vi "Global Variables.vi"() -> ()   [LabVIEW 2015]
uses:
  Arm Mode TypeDef.ctl
  Arm Notifier TypeDef.ctl
  Operator-Interface-Control-Board.git/trunk/LabVIEW/Analog_Input_TypeDef.ctl
  Operator-Interface-Control-Board.git/trunk/LabVIEW/Switch_Input_TypeDef.ctl
  Arm Mode LEDs.ctl
  IMU AHRS TypeDef.ctl
  Autonomous Mode.ctl
panel:
  in  "Arm Manual Angle":dbl
  in  "Autonomous Mode":T1
  out "Distance (cm)":dbl
  out "Arm Angle":dbl
  in  "Reset IMU":bool
  out "IMU Calibrated":bool
  in  "IMU AHRS":T2
  in  "Arm Mode LEDs":T3
  out "Air Pressure":dbl
  in  "Fire Ready":bool
  in  "Switch Inputs":T4
  out "Analog Inputs":T5
  in  "Arm Control":T6={"Arm Mode"=enum."Manual", "Manual Arm Angle"=0.0}
  in  "Current Arm Mode":T7=enum."Manual"
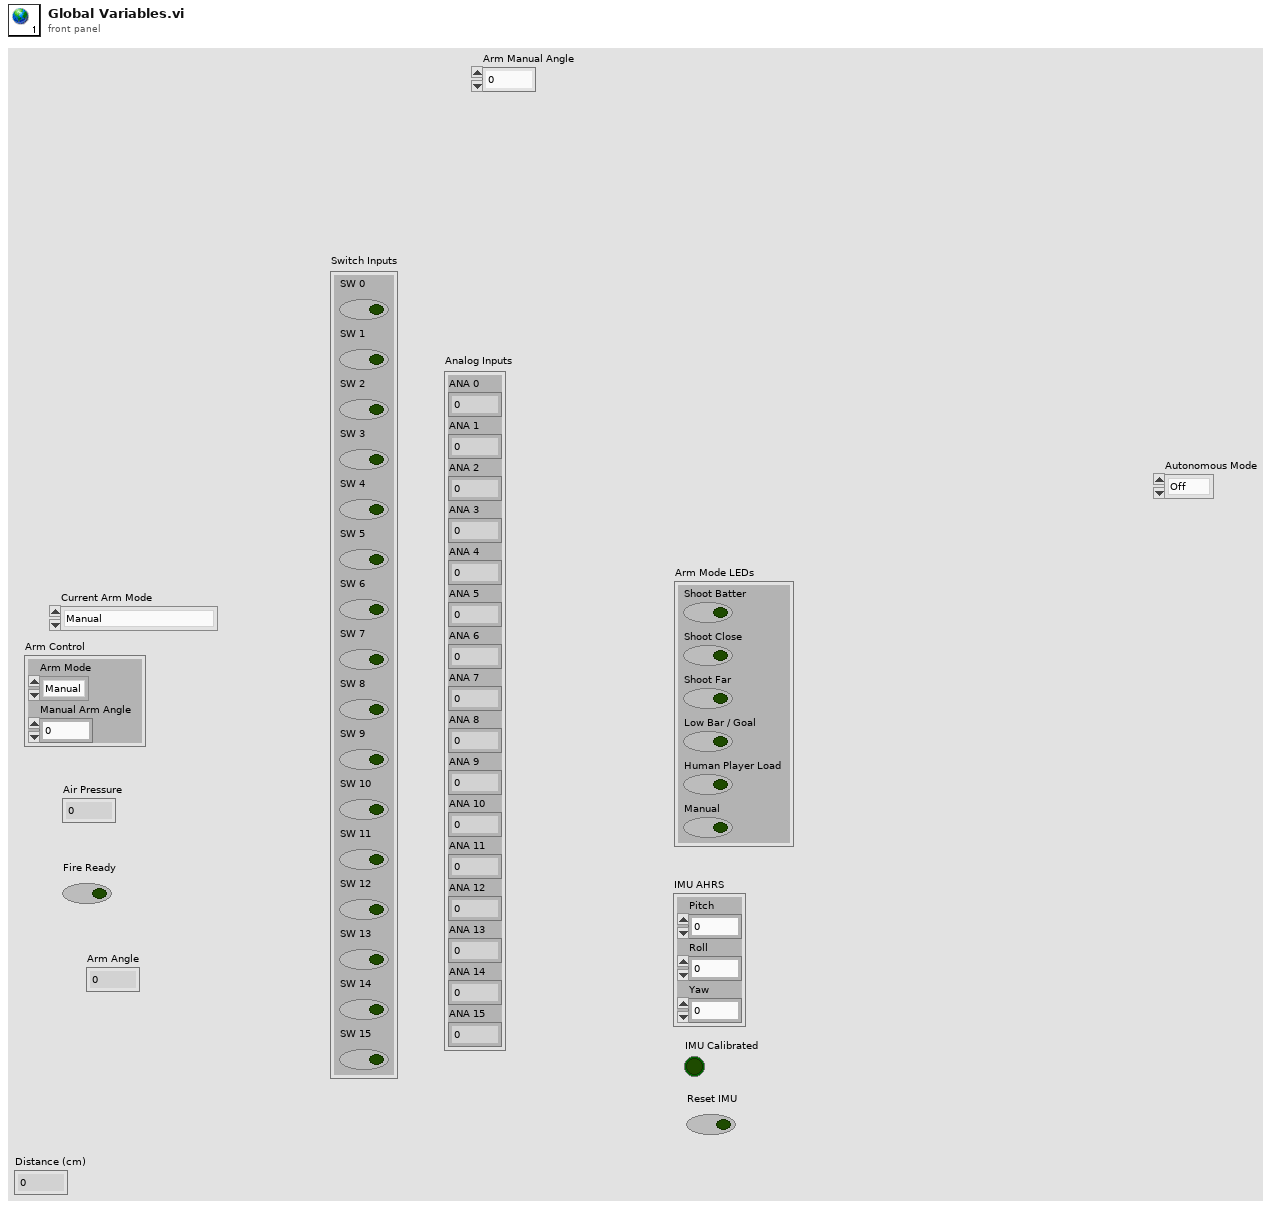
[diagram p1: front panel]
types:
  T1 = typedef "Autonomous Mode.ctl" = enum16{"Off", "Cross Defense", "Shoot A/B", "Shoot C/D", "Shoot E"}
  T2 = typedef "IMU AHRS TypeDef.ctl" = cluster{"Pitch":dbl, "Roll":dbl, "Yaw":dbl}
  T3 = typedef "Arm Mode LEDs.ctl" = cluster{"Shoot Batter":bool, "Shoot Close":bool, "Shoot Far":bool, "Low Bar / Goal":bool, "Human Player Load":bool, "Manual":bool}
  T4 = typedef "Switch_Input_TypeDef.ctl" = cluster{"SW 0":bool, "SW 1":bool, "SW 2":bool, "SW 3":bool, "SW 4":bool, "SW 5":bool, "SW 6":bool, "SW 7":bool, "SW 8":bool, "SW 9":bool, "SW 10":bool, "SW 11":bool, "SW 12":bool, "SW 13":bool, "SW 14":bool, "SW 15":bool}
  T5 = typedef "Analog_Input_TypeDef.ctl" = cluster{"ANA 0":u8, "ANA 1":u8, "ANA 2":u8, "ANA 3":u8, "ANA 4":u8, "ANA 5":u8, "ANA 6":u8, "ANA 7":u8, "ANA 8":u8, "ANA 9":u8, "ANA 10":u8, "ANA 11":u8, "ANA 12":u8, "ANA 13":u8, "ANA 14":u8, "ANA 15":u8}
  T6 = typedef "Arm Notifier TypeDef.ctl" = cluster{"Arm Mode":T7, "Manual Arm Angle":dbl}
  T7 = typedef "Arm Mode TypeDef.ctl" = enum16{"Unknown", "Disabled", "Locked", "Shoot Batter", "Shoot Close", "Cross Defense", "Human Player Load", "Low Bar / Goal", "Manual"}
diagram:
